vi "Alignment.vi"() -> ()   [LabVIEW 2016]
uses:
  Classes/Controller/Controller Folder/Controller.lvclass
panel:
  out "Sum":dbl[](array[numeric])=[1219.30639899585, 722.8896830877354, 52.864847366341415, 0.003106741190800654] format="%#_8g"
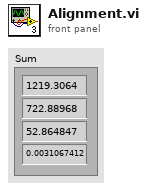
[diagram p1: front panel]
types:
  T1 = typedef "Controller.lvclass/Controllers.ctl" = cluster{"Copy of Motion.lvclass":refnum<class "Motion.lvclass">, "Copy of I-O.lvclass ":refnum<class "I-O.lvclass">, "Copy of Dispenser.lvclass":refnum<class "Dispenser.lvclass">}
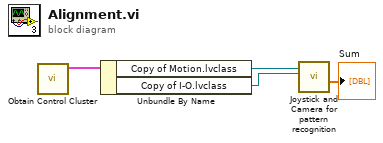
[diagram p0: block diagram]
diagram:
  n1 = call "Obtain Control Cluster.vi"() -> ("Control Out"=w3:T1)  [unwired: 11 in]
  n2 = Unbundle By Name(w3) -> ("Copy of Motion.lvclass"=w2:refnum<class "Motion.lvclass">, "Copy of I-O.lvclass"=w1:refnum<class "I-O.lvclass">)
  n3 = call "Joystick and Camera for pattern recognition.vi"("I-O in"=w1, "Motion in"=w2) -> ("Sum"=→"Sum":dbl[])  [unwired: 5 in, 2 out]
